vi "ejercicio 10 A.vi"() -> ()   [LabVIEW 2015]
panel:
  out "Raiz 1":dbl
  out "Raiz 2":dbl
  in  "Número C":dbl
  in  "Número A":dbl
  in  "Número B":dbl
  out "Discriminante":dbl
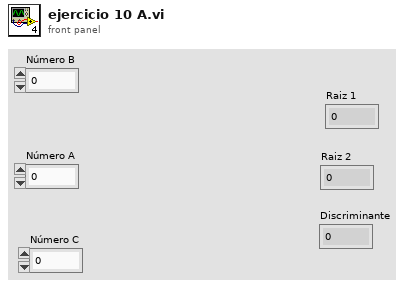
[diagram p1: front panel]
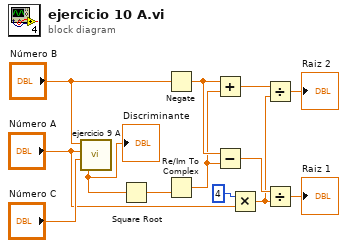
[diagram p0: block diagram]
diagram:
  n1 = call "ejercicio 9 A.vi"("Número C"="Número C", "Número A"="Número A", "Número B"="Número B") -> ("Discriminante"=w11:dbl)  [unwired: 3 out]
  "Discriminante" <- w11
  n2 = Square Root(x=w11) -> (sqrt(x)=w10:dbl)
  n3 = Negate(x="Número B") -> (-x=w8:dbl)
  n4 = Re/Im To Complex(1:w10) -> (0:w7:cdb)  [unwired: 1 in]
  n5 = Add(x=w8, y=w7) -> (x+y=w4:cdb)
  n6 = Subtract(x=w8, y=w7) -> (x-y=w6:cdb)
  n7 = Multiply(x=4, y="Número A") -> (x*y=w3:dbl)
  n8 = Divide(x=w4, y=w3) -> (x/y=→"Raiz 2":cdb)
  n9 = Divide(x=w6, y=w3) -> (x/y=→"Raiz 1":cdb)
